vi "endMission.vi"(8 "error in (no error)":errorcluster, 11 "GenericMission in":refnum<class "GenericMission.lvclass">) -> (0 "error out":errorcluster, 3 "GenericMission out":refnum<class "GenericMission.lvclass">)   [LabVIEW 2011, in "GenericMission.lvclass"]
uses:
  GenericMission.lvclass
  2 Globals/2 Message Logger.vi
  Logger/Logger.lvclass
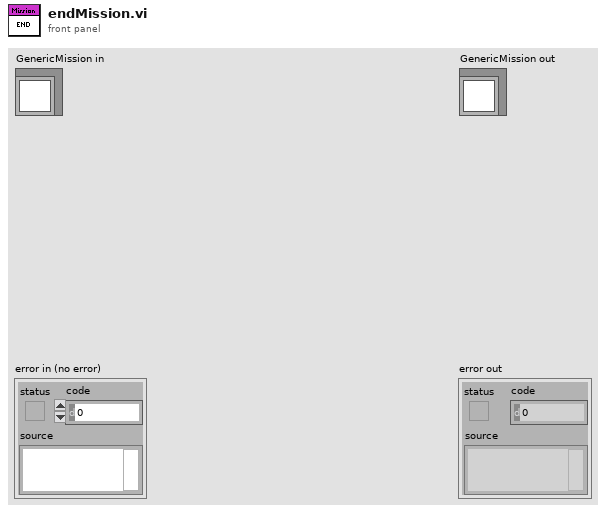
[diagram p1: front panel]
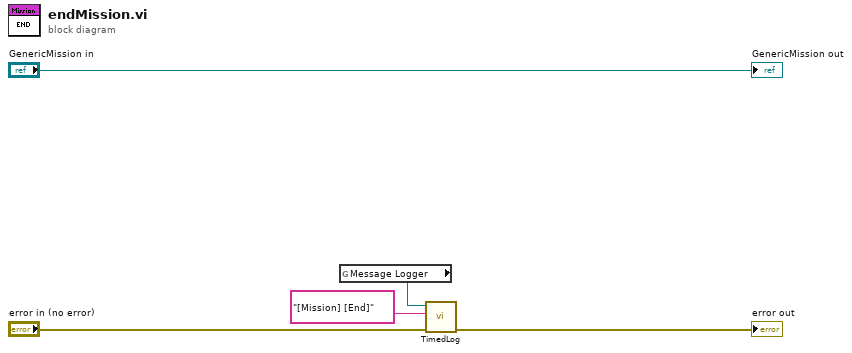
[diagram p0: block diagram]
diagram:
  n1 = global read "2 Message Logger.vi" "Message Logger"() -> (w3:refnum<class "Logger.lvclass">)
  n2 = call "TimedLog.vi"("error in (no error)"="error in (no error)", "Message"="[Mission] [End]", "Logger in"=w3) -> ("error out"=→"error out":errorcluster)  [unwired: 6 in, 2 out]
  "GenericMission out" <- "GenericMission in"
